vi "TEST-JSON-RPC.vi"() -> ()   [LabVIEW 2019]
uses:
  TEST-JSON-RPC--Cluster.ctl
  <vilib>/JDP Science/JSONtext/JSON Value Type.ctl
  <vilib>/numeric/Random Number (Range) DBL.vi
  <vilib>/numeric/Random Number (Range) I64.vi
  423c0946-e876-4033-917c-c4e0f5a656b4.vi
  ee9c883b-8f02-4ab6-8633-18d9b039323c.vi
  6f47a901-0ffd-4612-bb45-9ae4cf78a1c3.vi
  9d79f0c2-35ce-467d-8164-7d449b6aa026.vi
  53d3177d-6787-4563-b3f2-ec7d47ca270a.vi
  d9266a12-4538-4804-ad7c-12d0542650b7.vi
  <vilib>/numeric/sub_Random U32.vi
  <vilib>/JDP Science/JSONtext/JSON text to Variant (path).vi
  <vilib>/JDP Science/JSONtext/Find Item.vi
  <vilib>/JDP Science/JSONtext/Next JSON Value.vi
  <vilib>/JDP Science/JSONtext/String Subset.vi
  <vilib>/JDP Science/JSONtext/Parsing/Advance past next JSON Value (inlined COPY).vi
  <vilib>/JDP Science/JSONtext/Parsing/Advance past whitespace.vi
  <vilib>/JDP Science/JSONtext/Parsing/Advance past String.vi
  <vilib>/JDP Science/JSONtext/Parsing/Advance past Number.vi
  <vilib>/JDP Science/JSONtext/Parsing/Advance past Line Ending.vi
  <vilib>/JDP Science/JSONtext/JSON text to Variant.vi
  <vilib>/JDP Science/JSONtext/support/Format JSON Array Text.vi
  <vilib>/Utility/Data Type/Get Type Information.vi
  <vilib>/JDP Science/JSONtext/Parsing/Parse Full Path or Item Name.vi
  <vilib>/JDP Science/JSONtext/Parsing/Advance past Array.vi
  <vilib>/JDP Science/JSONtext/Parsing/Advance past Object.vi
  <vilib>/JDP Science/JSONtext/support/Error Cluster From Code.vi
  <vilib>/JDP Science/JSONtext/Offset/Find Item Locations by Path.vi
  JSON-RPC/JSON-RPC.lvclass
  <vilib>/JDP Science/JSONtext/LVClass Serializer/JSONtext LVClass Serializer.lvclass
  <vilib>/JDP Science/JSONtext/JSONtext.lvlib
  0ae8443b-0c4b-4e01-b233-50273e00e751.vi
panel:
  out "JSON Value Type":T1
  out "Names 3":string[](array[string])
  out "Params 3":string[](array[string])
  out "Clusters Section":dbl
  out "Arrays":dbl[](array[numeric])
  out "Clusters":T2
  out "Params 2":string[](array[string])
  out "Names 2":string[](array[string])
  out "Params":string[](array[string])
  out "Names":string[](array[string])
  out "REQ.Methods":string
  out "Match?":bool
  out "{JSON} Response":string
  out "{JSON} Requests":string
  out "4. parse response":dbl format="%#_6p"
  out "3. create response":dbl format="%#_6p"
  out "2. parse request":dbl format="%#_6p"
  out "1. create request":dbl format="%#_6p"
  out "REQ.Params":string
  out "results":string
  in  "Numeric":i32=3
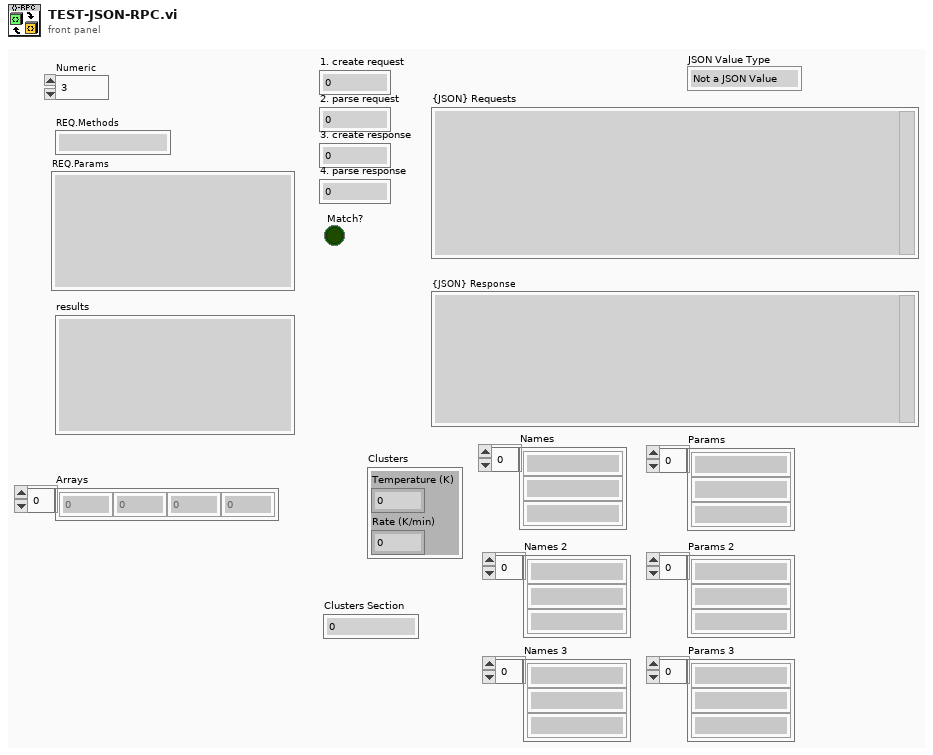
[diagram p1: front panel]
types:
  T1 = typedef "JSONtext.lvlib/JSON Value Type.ctl" = enum16{"Not a JSON Value", "JSON Object", "JSON Array", "String", "Number", "true", "false", "null"}
  T2 = typedef "TEST-JSON-RPC--Cluster.ctl" = cluster{"Temperature (K)":dbl, "Rate (K/min)":dbl}
  T3 = enum16{"Parse Error", "Invalid Request", "Method not found", "Invalid params", "Internal error", "Server error"}
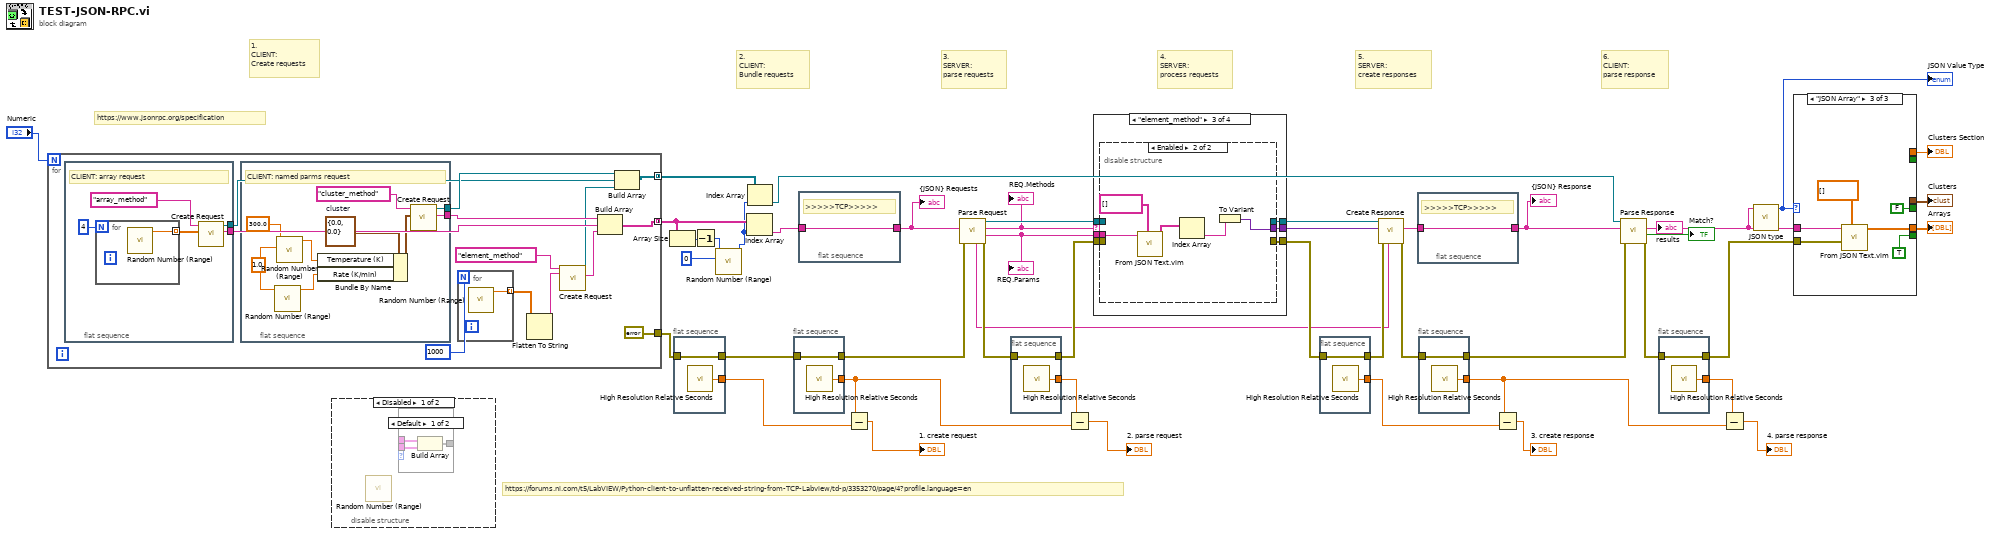
[diagram p0: block diagram]
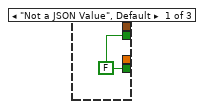
[diagram p2: hidden frame]
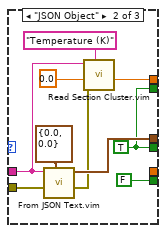
[diagram p3: hidden frame]
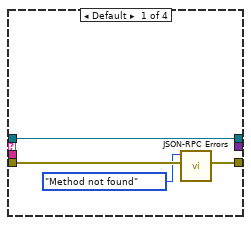
[diagram p4: hidden frame]
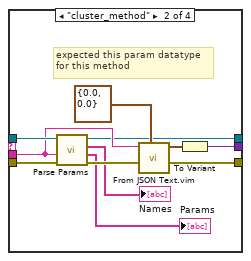
[diagram p5: hidden frame]
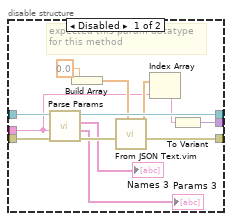
[diagram p6: hidden frame]
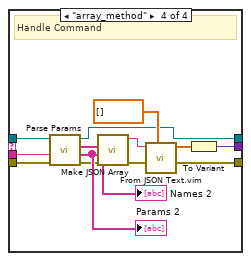
[diagram p7: hidden frame]
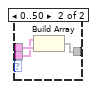
[diagram p8: hidden frame]
diagram:
  # "1.\nCLIENT:\nCreate requests"
  # "3.\nSERVER:\nparse requests"
  # "6.\nCLIENT:\nparse response"
  # "4.\nSERVER:\nprocess requests"
  # "5.\nSERVER:\ncreate responses"
  # "https://forums.ni.com/t5/LabVIEW/Python-client-to-unflatten-received-string-from-TCP-Labview/td-p/3353270/page/4?profile.language=en"
  # "2.\nCLIENT:\nBundle requests"
  # "https://www.jsonrpc.org/specification"
  n1 = for {
    N: "Numeric" -> [_]
    tunnel: [errorcluster {"status"=FALSE, "code"=0, "source"=""} ("error out")] -> w20
    tunnel: [w56] -> w9 mode=concatenating
    tunnel: [w52] -> w4 mode=concatenating
    n2 = flat-sequence {
      tunnel: [w73] -> w57
      tunnel: [w69] -> w49
      frame #0 {
        # "CLIENT: array request"
        n3 = for {
          N: 4 -> [_]
          tunnel: [w74] -> w70 mode=indexing
          n4 = call-poly <vilib>:"Random Number (Range).vi"() -> ("number"=w74:dbl)  [unwired: 11 in]
        }
        n5 = call "Create Request.vi"("params"=w70, "method"="array_method" ("Request.method")) -> ("{JSON} Requests"=w73:string, "JSON-RPC out"=w69:refnum<class "JSON-RPC.lvclass">)  [unwired: 6 in, 2 out]
      }
    }
    n6 = flat-sequence {
      tunnel: [w61] -> w55
      tunnel: [w60] -> w50
      frame #0 {
        w66 = 1.0 ("lower bound (0)")
        w68 = T2 {"Temperature (K)"=0.0, "Rate (K/min)"=0.0}  # cluster
        # "CLIENT: named parms request"
        n7 = call-poly <vilib>:"Random Number (Range).vi"("upper bound (100)"=w66) -> ("number"=w65:dbl)  [unwired: 10 in]
        n8 = call-poly <vilib>:"Random Number (Range).vi"("lower bound (0)"=w66, "upper bound (100)"=300.0 ("lower bound (0)")) -> ("number"=w64:dbl)  [unwired: 9 in]
        n9 = Bundle By Name(cluster=w68, "Temperature (K)"=w64, "Rate (K/min)"=w65) -> (w63:T2)
        n10 = call "Create Request.vi"("params"=w63, "method"="cluster_method" ("Request.method")) -> ("{JSON} Requests"=w61:string, "JSON-RPC out"=w60:refnum<class "JSON-RPC.lvclass">)  [unwired: 6 in, 2 out]
      }
    }
    n11 = for {
      N: 1000 -> [_]
      tunnel: [w59] -> w48 mode=indexing
      n12 = call-poly <vilib>:"Random Number (Range).vi"() -> ("number"=w59:dbl)  [unwired: 11 in]
    }
    n13 = Flatten To String(anything=w48) -> (data string=w47:string)  [unwired: 3 in, 2 out]
    n14 = call "Create Request.vi"("params"=w47, "method"="element_method" ("Request.method")) -> ("{JSON} Requests"=w54:string, "JSON-RPC out"=w51:refnum<class "JSON-RPC.lvclass">)  [unwired: 6 in, 2 out]
    n15 = Build Array(w55, w57, w54) -> (w56:string[])
    n16 = Build Array(w50, w49, w51) -> (w52:refnum<class "JSON-RPC.lvclass">[])
  }
  n17 = disable-structure shown="Disabled" {
    frame Disabled {
      n18 = call-poly <vilib>:"Random Number (Range).vi"() -> ()  [unwired: 11 in, 1 out]
      n19 = case shown="Default" {
        selector: _ -> [_ _]
        tunnel: _ -> [w77 w80]
        tunnel: _ -> [w76 w79]
        tunnel: [w75 w78] -> _
        frame Default {
          n20 = Build Array(w77, w76) -> (w75:void[])
        }
        frame 0..50 {
          n21 = Build Array(w79, w80) -> (w78:void[])
        }
      }
    }
    frame Enabled {
    }
  }
  n22 = Array Size(array=w9) -> (size(s)=w8:i32)
  n23 = flat-sequence {
    tunnel: [w81] -> w11
    tunnel: [w82] -> w44
    tunnel: w20 -> [w81]
    frame #0 {
      n24 = call <vilib>:"High Resolution Relative Seconds.vi"() -> ("relative seconds"=w82:dbl)
    }
  }
  n25 = Decrement(x=w8) -> (x-1=w5:i32)
  n26 = call-poly <vilib>:"Random Number (Range).vi"("lower bound (-100)"=i64 0, "upper bound (100)"=w5) -> ("number"=w2:i64)  [unwired: 9 in]
  n27 = Index Array(array=w9, index=w2) -> (element=w10:string)
  n28 = Index Array(array=w4, index=w2) -> (element=w3:refnum<class "JSON-RPC.lvclass">)
  n29 = flat-sequence {
    tunnel: [w83] -> w29
    tunnel: [w84] -> w42
    tunnel: w11 -> [w83]
    frame #0 {
      n30 = call <vilib>:"High Resolution Relative Seconds.vi"() -> ("relative seconds"=w84:dbl)
    }
  }
  n31 = flat-sequence {
    tunnel: w10 -> [w85]
    tunnel: [w85] -> w27
    frame #0 {
      # ">>>>>TCP>>>>>"
    }
  }
  n32 = Subtract(x=w42, y=w44) -> (x-y=→"1. create request":dbl)
  n33 = call "Parse Request.vi"("error in (no error)"=w29, "{JSON} Request"=w27) -> ("error out"=w28:errorcluster, "Params"=w12:string, "Method"=w13:string, "JSON-RPC out"=w31:refnum<class "JSON-RPC.lvclass">, "ID"=w14:string)  [unwired: 5 in]
  "REQ.Params" <- w12
  "REQ.Methods" <- w13
  n34 = flat-sequence {
    tunnel: [w86] -> w43
    tunnel: [w87] -> w39
    tunnel: w28 -> [w86]
    frame #0 {
      n35 = call <vilib>:"High Resolution Relative Seconds.vi"() -> ("relative seconds"=w87:dbl)
    }
  }
  n36 = Subtract(x=w39, y=w42) -> (x-y=→"2. parse request":dbl)
  n37 = case shown="\"element_method\"" w13 {
    tunnel: w43 -> [w91 w97 w106 w136]
    tunnel: [w90 w102 w108 w127] -> w40
    tunnel: [_ w101 w107 w138] -> w19
    tunnel: w12 -> [_ w95 w103 w135]
    tunnel: w31 -> [w88 w96 w105 w137]
    tunnel: [w88 w94 w104 w126] -> w30
    frame Default {
      n38 = call "JSON-RPC Errors.vi"("error in"=w91, "Enum"=T3."Method not found") -> ("error out"=w90:errorcluster)  [unwired: 9 in]
    }
    frame "cluster_method" {
      # "expected this param datatype\nfor this method"
      n39 = call "Parse Params.vi"("error in (no error)"=w97, "{JSON} Params"=w95, "JSON-RPC in"=w96) -> ("error out"=w98:errorcluster, "Params"=→"Params":string[], "Names"=→"Names":string[], "JSON-RPC out"=w94:refnum<class "JSON-RPC.lvclass">)  [unwired: 5 in]
      n40 = call "From JSON Text.vim"("Data Type and Default Value"=T2 {"Temperature (K)"=0.0, "Rate (K/min)"=0.0} ("Cluster"), "error in (no error)"=w98, "JSON"=w95) -> ("error out"=w102:errorcluster, "Data out"=w99:T2)  [unwired: 7 in]
      n41 = To Variant(anything=w99) -> (Variant=w101:variant)
    }
    frame "element_method" {
      n42 = disable-structure shown="Enabled" {
        disable-tunnel: [w120 _] -> w108
        disable-tunnel: [w119 w121] -> w107
        disable-tunnel: w106 -> [w117 _]
        disable-tunnel: w105 -> [w116 _]
        disable-tunnel: [w115 _] -> w104
        disable-tunnel: w103 -> [w109 w125]
        frame Disabled {
          # "expected this param datatype\nfor this method"
          n43 = call "Parse Params.vi"("error in (no error)"=w117, "{JSON} Params"=w109, "JSON-RPC in"=w116) -> ("error out"=w118:errorcluster, "Params"=→"Params 3":string[], "Names"=→"Names 3":string[], "JSON-RPC out"=w115:refnum<class "JSON-RPC.lvclass">)  [unwired: 5 in]
          n44 = Build Array(0.0) -> (w110:dbl[])
          n45 = call "From JSON Text.vim"("Data Type and Default Value"=w110, "error in (no error)"=w118) -> ("error out"=w120:errorcluster, "Data out"=w111:dbl[])  [unwired: 8 in]
          n46 = Index Array(array=w111) -> ()  [unwired: 1 in, 1 out]
          n47 = To Variant(anything=w109) -> (Variant=w119:variant)
        }
        frame Enabled {
          n48 = call "From JSON Text.vim"("Data Type and Default Value"=string[] [], "JSON"=w125) -> ("Data out"=w123:string[])  [unwired: 8 in, 1 out]
          n49 = Index Array(array=w123) -> (element=w122:string)  [unwired: 1 in]
          n50 = To Variant(anything=w122) -> (Variant=w121:variant)
        }
      }
    }
    frame "array_method" {
      # "Handle Command"
      n51 = call "Parse Params.vi"("error in (no error)"=w136, "{JSON} Params"=w135, "JSON-RPC in"=w137) -> ("error out"=w128:errorcluster, "Params"=w130:string[], "Names"=→"Names 2":string[], "JSON-RPC out"=w126:refnum<class "JSON-RPC.lvclass">)  [unwired: 5 in]
      "Params 2" <- w130
      n52 = call <vilib>:"Make JSON Array.vi"("error in (no error)"=w128, "JSON Elements"=w130) -> ("error out"=w129:errorcluster, "<JSON>"=w131:string)  [unwired: 8 in]
      n53 = call "From JSON Text.vim"("Data Type and Default Value"=dbl[] [], "error in (no error)"=w129, "JSON"=w131) -> ("error out"=w127:errorcluster, "Data out"=w133:dbl[])  [unwired: 7 in]
      n54 = To Variant(anything=w133) -> (Variant=w138:variant)
    }
  }
  n55 = flat-sequence {
    tunnel: [w139] -> w22
    tunnel: [w140] -> w37
    tunnel: w40 -> [w139]
    frame #0 {
      n56 = call <vilib>:"High Resolution Relative Seconds.vi"() -> ("relative seconds"=w140:dbl)
    }
  }
  n57 = call "Create Response.vi"("id"=w14, "error in (no error)"=w22, "result"=w19, "JSON-RPC in"=w30) -> ("error out"=w21:errorcluster, "{JSON} Response"=w26:string)  [unwired: 5 in, 1 out]
  n58 = flat-sequence {
    tunnel: w26 -> [w141]
    tunnel: [w141] -> w23
    frame #0 {
      # ">>>>>TCP>>>>>"
    }
  }
  n59 = flat-sequence {
    tunnel: [w142] -> w25
    tunnel: [w143] -> w35
    tunnel: w21 -> [w142]
    frame #0 {
      n60 = call <vilib>:"High Resolution Relative Seconds.vi"() -> ("relative seconds"=w143:dbl)
    }
  }
  n61 = Subtract(x=w35, y=w37) -> (x-y=→"3. create response":dbl)
  n62 = call "Parse Response.vi"("error in (no error)"=w25, "{JSON} Response"=w23, "JSON-RPC in"=w3) -> ("error out"=w24:errorcluster, "Equal?"=→"Match?":bool, "results"=w7:string)  [unwired: 4 in, 2 out]
  "results" <- w7
  n63 = flat-sequence {
    tunnel: [w144] -> w18
    tunnel: [w145] -> w36
    tunnel: w24 -> [w144]
    frame #0 {
      n64 = call <vilib>:"High Resolution Relative Seconds.vi"() -> ("relative seconds"=w145:dbl)
    }
  }
  n65 = Subtract(x=w36, y=w35) -> (x-y=→"4. parse response":dbl)
  n66 = call <vilib>:"JSON type.vi"("JSON"=w7) -> ("JSON Value Type"=w1:T1)  [unwired: 9 in, 1 out]
  "JSON Value Type" <- w1
  n67 = case shown="\"JSON Array\"" w1 {
    tunnel: w7 -> [_ w152 w162]
    tunnel: w18 -> [_ w155 w161]
    tunnel: [_ _ w159] -> w16
    tunnel: [w146 FALSE TRUE] -> _
    tunnel: [_ w154 _] -> w17
    tunnel: [w146 w148 FALSE] -> _
    tunnel: [_ w149 _] -> w15
    tunnel: [_ w148 _] -> _
    frame "Not a JSON Value", Default {
      w146 = FALSE
    }
    frame "JSON Object" {
      w148 = TRUE
      n68 = call "From JSON Text.vim"("Data Type and Default Value"=T2 {"Temperature (K)"=0.0, "Rate (K/min)"=0.0} ("Cluster"), "error in (no error)"=w155, "JSON"=w152) -> ("error out"=w147:errorcluster, "Data out"=w154:T2)  [unwired: 7 in]
      n69 = call "Read Section Cluster.vim"("Section (Cluster Name)"="Temperature (K)", "error in (no error)"=w147, "Section Cluster"=0.0, "JSON Sections"=w152) -> ("Cluster set from section"=w149:dbl)  [unwired: 4 in, 2 out]
    }
    frame "JSON Array" {
      n70 = call "From JSON Text.vim"("Data Type and Default Value"=dbl[] [], "error in (no error)"=w161, "JSON"=w162) -> ("Data out"=w159:dbl[])  [unwired: 7 in, 1 out]
    }
  }
  "Clusters" <- w17
  "Arrays" <- w16
  "Clusters Section" <- w15
  "{JSON} Requests" <- w27
  "{JSON} Response" <- w23
